vi "CAN Write data.vi"(8 "error in (no error)":errorcluster, 10 "data":dbl[](array[numeric]), 11 "WRITE DATA":T1[](array[typedef])) -> (0 "error out":errorcluster)   [LabVIEW 2018]
uses:
  Controls/READ CAN CLUSTER.ctl
  <vilib>/xnet/xnet.llb/XNET Create Session (Signal Output Single-point).vi
  <vilib>/xnet/xnet.llb/XNET Write (Signal Single-point).vi
panel:
  in  "CAN SIGNAL":string
  out "session out 2":refnum<k21>
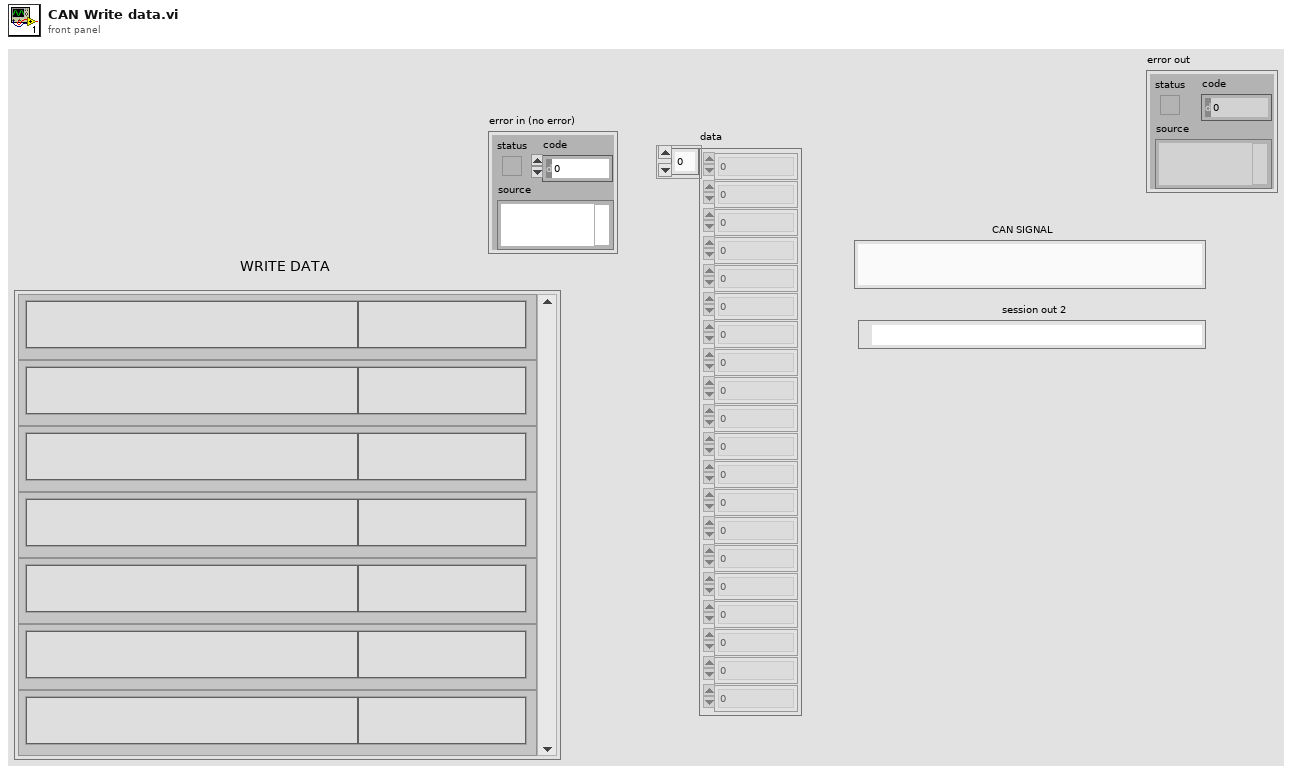
[diagram p1: front panel]
types:
  T1 = typedef "READ CAN CLUSTER.ctl" = cluster{"FUNCTION":string, "DATA":string}
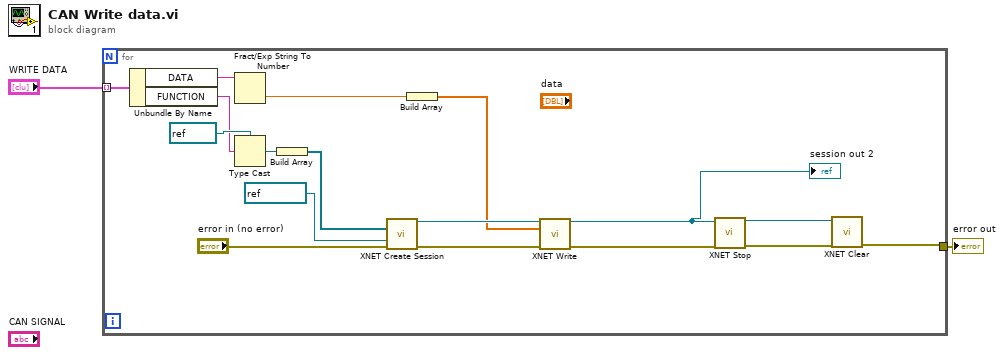
[diagram p0: block diagram]
diagram:
  n1 = for {
    tunnel: [w4] -> w2
    tunnel: "WRITE DATA" -> [w12] mode=indexing
    n2 = Unbundle By Name(w12) -> ("DATA"=w10:string, "FUNCTION"=w11:string)
    n3 = Fract/Exp String To Number(string=w10) -> (number=w9:dbl)  [unwired: 3 in, 1 out]
    n4 = Type Cast(type=refnum<k21> " " ("XNET Signal"), x=w11) -> (*(type *) &x=w17:refnum<k21>)
    n5 = Build Array(w17) -> (w13:refnum<k21>[])
    n6 = call-poly <vilib>:"XNET Create Session.vi"("signal list"=w13, "interface"=refnum<k21> "CAN1" ("Select Interface"), "error in (no error)"="error in (no error)") -> ("session out"=w15:refnum<k21>, "error out"=w14:errorcluster)  [unwired: 11 out]
    n7 = Build Array(w9) -> (w8:dbl[])
    n8 = call-poly <vilib>:"XNET Write.vi"("session in"=w15, "data"=w8, "error in (no error)"=w14) -> ("session out"=w3:refnum<k21>, "error out"=w6:errorcluster)  [unwired: 11 in]
    "session out 2" <- w3
    n9 = call <vilib>:"XNET Stop.vi"("session in"=w3, "error in (no error)"=w6) -> ("session out"=w7:refnum<k21>, "error out"=w5:errorcluster)  [unwired: 12 in]
    n10 = call <vilib>:"XNET Clear.vi"("session in"=w7, "error in (no error)"=w5) -> ("error out"=w4:errorcluster)  [unwired: 13 in]
  }
  "error out" <- w2
